vi "Settings Dialog.vi"(8 "error in (no error)":errorcluster, 11 "Settings in":T2) -> (0 "error out":errorcluster, 1 "Cancelled?":bool, 2 "UI Refresh Needed?":bool, 3 "Settings out":T2)   [LabVIEW 2013, in "AvaSpec Settings.lvlib"]
doc: "Dialog for selecting user specified settings."
uses:
  AvaSpec Settings.lvlib
  Settings.ctl
  Acquisition/Hardware Configuration.ctl
  Libraries/AS-5216-DLL/AVS settings.ctl
  Acquisition/Sphere Indicator.ctl
  Logging/Logging Configuration.ctl
  <vilib>/Utility/xml.llb/Write to XML File(string).vi
  Acquisition/AvaSpec Acquisition.lvlib
  Logging/AvaSpec Logging.lvlib
  Libraries/IRRAD-DLL/AVSirrad.lvlib
panel:
  in  "Sphere Indicator":T1
  in  "Number Measurements to Average":u32=1
  in  "Integration Time (ms)":sgl=100.0
  in  "Calibration File Path":path
  in  "Aux Correction File Path":path
  in  "Log File Path":path
  in  "Cancel Button":bool
  in  "OK Button":bool
  # "Non visible portion of dialog (needed for connector pane)."
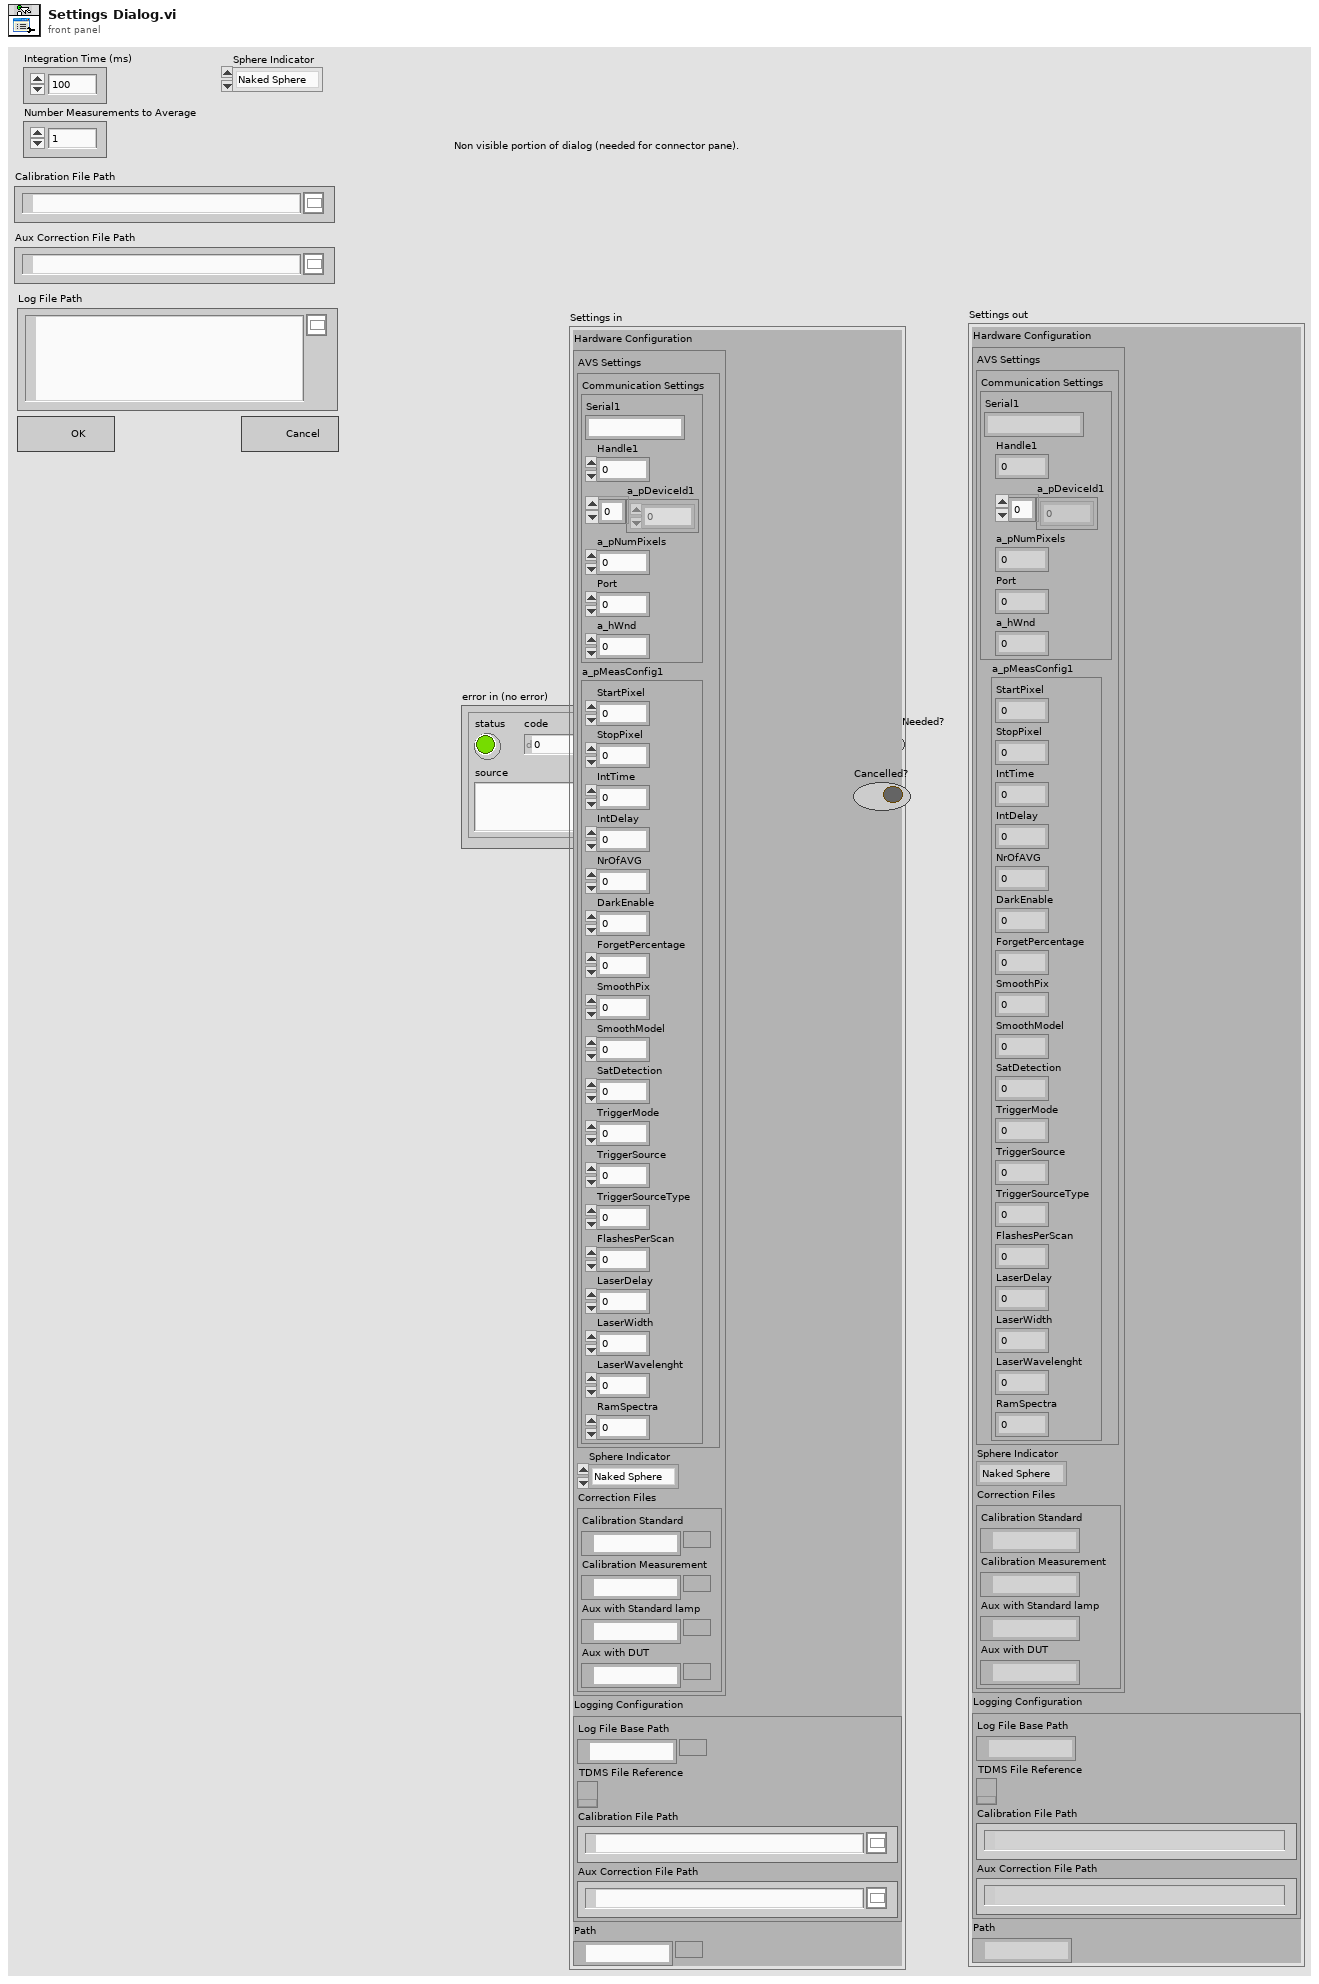
[diagram p1: front panel]
types:
  T1 = typedef "Sphere Indicator.ctl" = enum16{"Naked Sphere", "Insulated Sphere"}
  T2 = typedef "AvaSpec Settings.lvlib/Settings.ctl" = cluster{"Hardware Configuration":T3, "Logging Configuration":T5, "Path":path}
  T3 = typedef "AvaSpec Acquisition.lvlib/Hardware Configuration.ctl" = cluster{"AVS Settings":T4, "Sphere Indicator":T1, "Correction Files":cluster{"Calibration Standard":path, "Calibration Measurement":path, "Aux with DUT":path, "Aux with Standard lamp":path}}
  T4 = typedef "AVSirrad.lvlib/AVS settings.ctl" = cluster{"Communication Settings":cluster{"Serial1":string, "Handle1":i32, "a_pDeviceId1":u8[], "a_pNumPixels":u16, "Port":i32, "a_hWnd":i32}, "a_pMeasConfig1":cluster{"StartPixel":u16, "StopPixel":u16, "IntTime":sgl, "IntDelay":u32, "NrOfAVG":u32, "DarkEnable":u8, "ForgetPercentage":u8, "SmoothPix":u16, "SmoothModel":u8, "SatDetection":u8, "TriggerMode":u8, "TriggerSource":u8, "TriggerSourceType":u8, "FlashesPerScan":u16, "LaserDelay":u32, "LaserWidth":u32, "LaserWavelenght":sgl, "RamSpectra":u16}}
  T5 = typedef "AvaSpec Logging.lvlib/Logging Configuration.ctl" = cluster{"Log File Base Path":path, "TDMS File Reference":refnum<k34>, "Calibration File Path":path, "Aux Correction File Path":path}
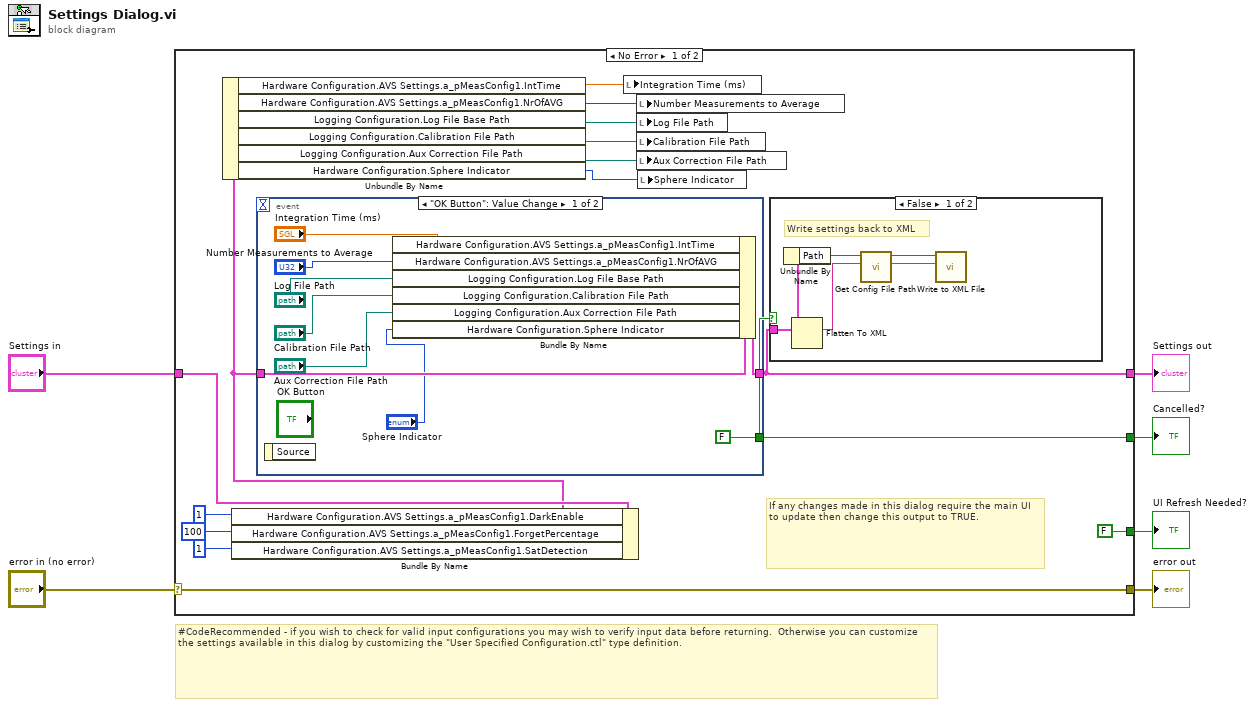
[diagram p0: block diagram]
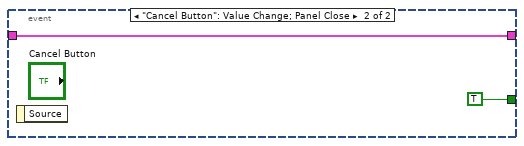
[diagram p3: hidden frame]
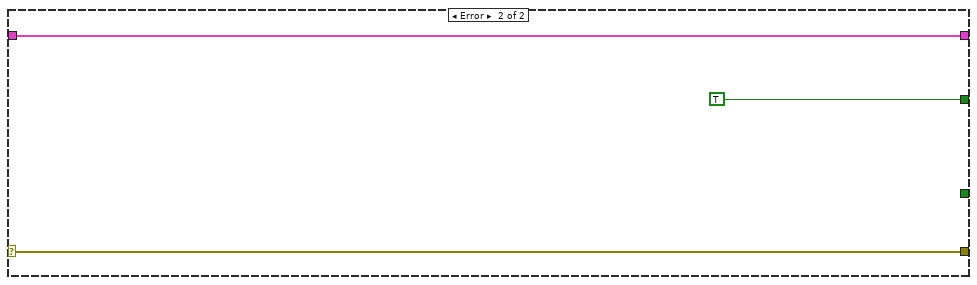
[diagram p4: hidden frame]
diagram:
  # "#CodeRecommended - if you wish to check for valid input configurations you may wish to verify input data before returning.  Otherwise you can customize the settings available in this dialog by customizing the \"User Specified Configuration.ctl\" type definition."
  n1 = case shown="No Error" "error in (no error)" {
    selector: "error in (no error)" -> [w21 w39]
    tunnel: [w21 w39] -> w5
    tunnel: "Settings in" -> [w12 w38]
    tunnel: [w18 w38] -> w3
    tunnel: [FALSE ("UI Refresh Needed?") _] -> w2
    tunnel: [w19 TRUE ("UI Refresh Needed?")] -> w1
    frame No Error {
      # "If any changes made in this dialog require the main UI to update then change this output to TRUE."
      n2 = Bundle By Name(cluster=w12, "Hardware Configuration.AVS Settings.a_pMeasConfig1.DarkEnable"=u8 1 ("Hardware Configuration.a_pMeasConfig1.DarkEnable"), "Hardware Configuration.AVS Settings.a_pMeasConfig1.ForgetPercentage"=u8 100 ("Hardware Configuration.a_pMeasConfig1.SatDetection"), "Hardware Configuration.AVS Settings.a_pMeasConfig1.SatDetection"=u8 1 ("Hardware Configuration.a_pMeasConfig1.SatDetection")) -> (w11:T2)
      n3 = Unbundle By Name(w11) -> ("Hardware Configuration.AVS Settings.a_pMeasConfig1.IntTime"=w17:sgl, "Hardware Configuration.AVS Settings.a_pMeasConfig1.NrOfAVG"=w15:u32, "Logging Configuration.Log File Base Path"=w16:path, "Logging Configuration.Calibration File Path"=w14:path, "Logging Configuration.Aux Correction File Path"=w13:path, "Hardware Configuration.Sphere Indicator"=w7:T1)
      n4 = event shown="[0] \"OK Button\": Value Change" {
        selector: _ -> [_ _]
        dyn-events: _ -> [_ _]
        timeout: _ -> [_ _]
        tunnel: [w32 w36] -> w18
        tunnel: w11 -> [w33 w36]
        tunnel: [FALSE ("UI Refresh Needed?") TRUE ("UI Refresh Needed?")] -> w19
        event "OK Button": Value Change {
          n5 = event-data() -> ()  [unwired: 1 in, 1 out]
          n6 = Bundle By Name(cluster=w33, "Hardware Configuration.AVS Settings.a_pMeasConfig1.IntTime"="Integration Time (ms)", "Hardware Configuration.AVS Settings.a_pMeasConfig1.NrOfAVG"="Number Measurements to Average", "Logging Configuration.Log File Base Path"="Log File Path", "Logging Configuration.Calibration File Path"="Calibration File Path", "Logging Configuration.Aux Correction File Path"="Aux Correction File Path", "Hardware Configuration.Sphere Indicator"="Sphere Indicator") -> (w32:T2)
        }
        event "Cancel Button": Value Change; Panel Close {
          n7 = event-data() -> ()  [unwired: 1 in, 1 out]
        }
      }
      n8 = local write "Integration Time (ms)"(w17) -> ()
      n9 = local write "Number Measurements to Average"(w15) -> ()
      n10 = local write "Log File Path"(w16) -> ()
      n11 = local write "Calibration File Path"(w14) -> ()
      n12 = local write "Aux Correction File Path"(w13) -> ()
      n13 = local write "Sphere Indicator"(w7) -> ()
      n14 = case shown="False" w19 {
        tunnel: w18 -> [w23 _]
        frame False {
          # "Write settings back to XML"
          n15 = Unbundle By Name(w23) -> ("Path"=w22:path)
          n16 = Flatten To XML(anything=w23) -> (xml string=w24:string)
          n17 = call "Get Config File Path.vi"("Path"=w22) -> ("XML File Path"=w25:path)  [unwired: 9 in, 1 out]
          n18 = call-poly <vilib>:"Write to XML File.vi"("XML Input"=w24, "XML File Path"=w25) -> ()  [unwired: 7 in, 3 out]
        }
        frame True {
        }
      }
    }
    frame Error {
    }
  }
  "UI Refresh Needed?" <- w2
  "error out" <- w5
  "Settings out" <- w3
  "Cancelled?" <- w1
